vi "GE5565 Open (Cluster) mod.vi"(4 "error in (no error)":errorcluster, 6 "VISA resource name (empty)":refnum<visa-resource-name>, 7 "device (1)":i32=1) -> (0 "error out":errorcluster {"code" format="%.0x"}, 3 "VMIC-5565":T1)   [LabVIEW 2019, in "RefMem DMA Engine.lvlib"]
doc: "Opens a reference to the specified IRIG device and sets the IRIG configuration to defaults:\n\ntime code format: IRIG B\nexternal time-code carrier enabled: FALSE\ninternal sync enabled: FALSE"
uses:
  RefMem DMA Engine.lvlib
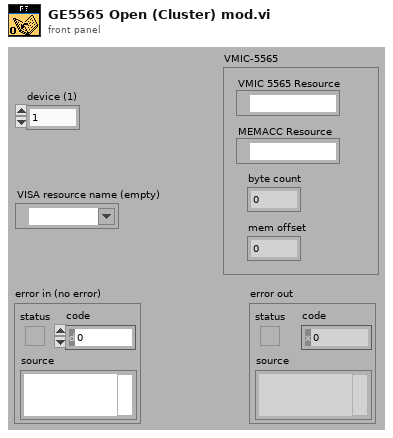
[diagram p1: front panel]
types:
  T1 = cluster{"VMIC 5565 Resource":refnum<visa-resource-name>, "MEMACC Resource":refnum<visa-resource-name>, "byte count":u32, "mem offset":u32}
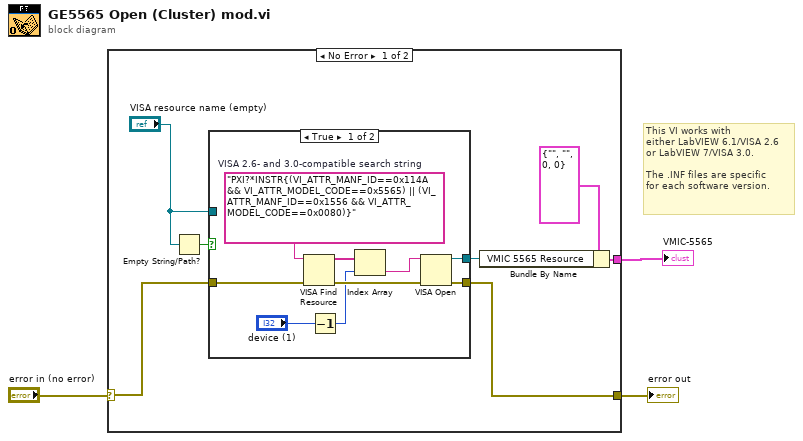
[diagram p0: block diagram]
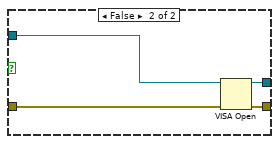
[diagram p2: hidden frame]
diagram:
  # "This VI works with\neither LabVIEW 6.1/VISA 2.6 \nor LabVIEW 7/VISA 3.0.\n\nThe .INF files are specific\nfor each software version."
  n1 = case shown="No Error" "error in (no error)" {
    selector: "error in (no error)" -> [w10 w24]
    tunnel: [w9 w24] -> w2
    tunnel: [w4 _] -> w1
    frame No Error {
      n2 = Empty String/Path?(string/path="VISA resource name (empty)") -> (empty?=w8:bool)
      n3 = case shown="True" w8 {
        tunnel: w10 -> [w18 w21]
        tunnel: [w12 w23] -> w9
        tunnel: [w11 w22] -> w5
        tunnel: "VISA resource name (empty)" -> [_ w20]
        frame True {
          w19 = "PXI?*INSTR{(VI_ATTR_MANF_ID==0x114A && VI_ATTR_MODEL_CODE==0x5565) || (VI_ATTR_MANF_ID==0x1556 && VI_ATTR_MODEL_CODE==0x0080)}"  # VISA 2.6- and 3.0-compatible search string
          n4 = VISA Find Resource(8:w18, 11:w19) -> (0:w17:errorcluster, 3:w16:string[])  [unwired: 2 out]
          n5 = Decrement(x="device (1)") -> (x-1=w13:i32)
          n6 = Index Array(array=w16, index=w13) -> (element=w14:string)
          n7 = VISA Open(error in (no error)=w17, VISA resource name=w14) -> (VISA resource name=w11:refnum<visa-resource-name>, error out=w12:errorcluster)  [unwired: 3 out]
        }
        frame False {
          n8 = VISA Open(error in (no error)=w21, VISA resource name=w20) -> (VISA resource name=w22:refnum<visa-resource-name>, error out=w23:errorcluster)  [unwired: 3 out]
        }
      }
      n9 = Bundle By Name(cluster=T1 {"VMIC 5565 Resource"="", "MEMACC Resource"="", "byte count"=0, "mem offset"=0} ("VMIC-5565"), "VMIC 5565 Resource"=w5) -> (w4:T1)
    }
    frame Error {
    }
  }
  "error out" <- w2
  "VMIC-5565" <- w1
